vi "divide.vi"   [LabVIEW 2023, in "LabGRAD.lvlib" / "Value.lvclass"]
uses:
  Value.lvclass
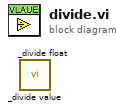
[diagram p0: block diagram]
diagram:
  n1 = call "_divide value.vi"() -> ()  [unwired: 9 in, 3 out]
  n2 = call "_divide float.vi"() -> ()  [unwired: 9 in, 3 out]
